vi "hc.vi"(9 "hcUse":string="VARS", 10 "modelName":string="VVV", 11 "Data":dbl[][](array[numeric])) -> ()   [LabVIEW 2014]
uses:
  <vilib>/Analysis/NI_AALBase.lvlib
  <vilib>/Analysis/baseanly.llb/Real A x B.vi
  <vilib>/Analysis/Matrix/NI_Matrix.lvlib
  <vilib>/Analysis/Matrix/Numeric/Conversions/Matrix To Array - RM.vi
  <vilib>/gmath/NI_Gmath.lvlib
panel:
  out "hcPairs":dbl[][](array[numeric])
  in  "Possible Use Names":string[](array[string])=["VARS", "STD", "SPH", "PCS", "PCR", "SVD"]
  in  "Possible Model Names":string[](array[string])=["E", "V", "EII", "VII", "EEE", "VVV"]
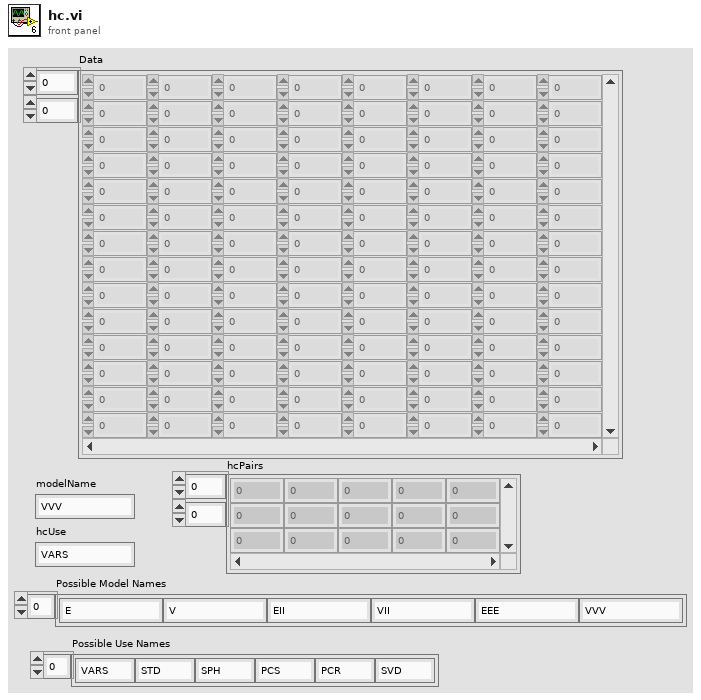
[diagram p1: front panel]
types:
  T1 = typedef "NI_Matrix.lvlib/RealMatrix.ctl" = dbl[][]
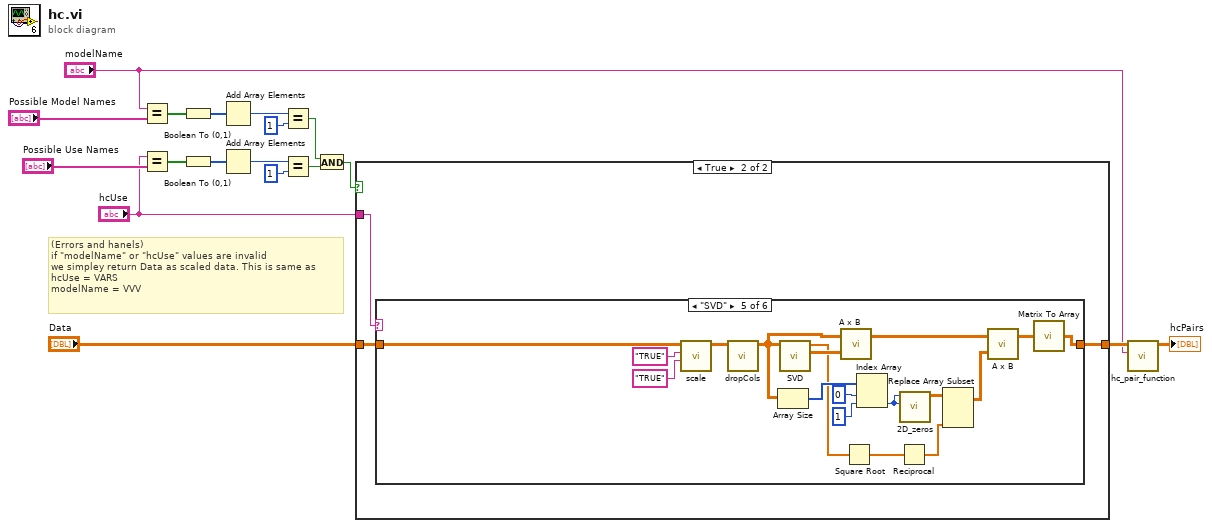
[diagram p0: block diagram]
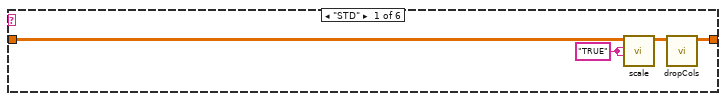
[diagram p3: hidden frame]
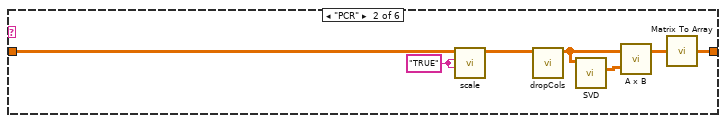
[diagram p4: hidden frame]
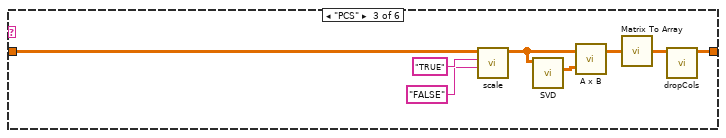
[diagram p5: hidden frame]
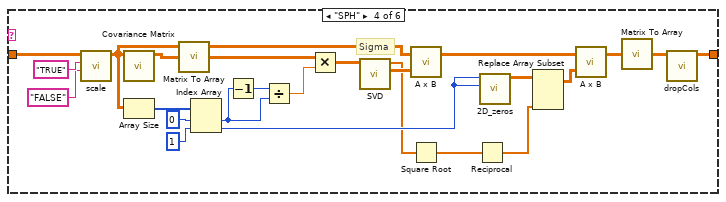
[diagram p6: hidden frame]
diagram:
  # "(Errors and hanels)\nif \"modelName\" or \"hcUse\" values are invalid\nwe simpley return Data as scaled data. This is same as\nhcUse = VARS\nmodelName = VVV"
  n1 = Equal?(x="modelName", y="Possible Model Names") -> (x = y?=w17:bool[])
  n2 = Equal?(x="hcUse", y="Possible Use Names") -> (x = y?=w14:bool[])
  n3 = Boolean To (0,1)(Boolean=w17) -> (0, 1=w16:i16[])
  n4 = Boolean To (0,1)(Boolean=w14) -> (0, 1=w15:i16[])
  n5 = Add Array Elements(numeric array=w16) -> (sum=w12:i16)
  n6 = Add Array Elements(numeric array=w15) -> (sum=w10:i16)
  n7 = Equal?(x=w12, y=i16 1) -> (x = y?=w8:bool)
  n8 = Equal?(x=w10, y=i16 1) -> (x = y?=w7:bool)
  n9 = And(x=w8, y=w7) -> (x .and. y?=w6:bool)
  n10 = case shown="True" w6 {
    tunnel: "Data" -> [w19 w21]
    tunnel: [w19 w20] -> w3
    tunnel: "hcUse" -> [_ w22]
    frame False {
    }
    frame True {
      n11 = case shown="\"SVD\"" w22 {
        tunnel: w21 -> [w26 w33 w38 w65 w68 w84]
        tunnel: [w23 w28 w36 w42 w66 w84] -> w20
        frame "STD" {
          w25 = "TRUE" ("Center")
          n12 = call "scale.vi"("Scale"=w25, "Center"=w25, "data"=w26) -> ("data (scaled)"=w24:dbl[][])  [unwired: 8 in]
          n13 = call "dropCols.vi"("data"=w24) -> ("data (columns dropped)"=w23:dbl[][])  [unwired: 10 in]
        }
        frame "PCR" {
          w32 = "TRUE" ("Center")
          n14 = call "scale.vi"("Scale"=w32, "Center"=w32, "data"=w33) -> ("data (scaled)"=w31:dbl[][])  [unwired: 8 in]
          n15 = call "dropCols.vi"("data"=w31) -> ("data (columns dropped)"=w27:dbl[][])  [unwired: 10 in]
          n16 = call "SVD.vi"("data (scaled)"=w27) -> ("v"=w30:dbl[][])  [unwired: 9 in, 1 out]
          n17 = call-poly <vilib>:"A x B.vi"("B"=w30, "A"=w27) -> ("A x B"=w29:T1)  [unwired: 1 out]
          n18 = call-poly <vilib>:"Matrix To Array.vi"("Real Matrix"=w29) -> ("Real 2D Array"=w28:dbl[][])
        }
        frame "PCS" {
          n19 = call "scale.vi"("Scale"="FALSE" ("Center"), "Center"="TRUE", "data"=w38) -> ("data (scaled)"=w40:dbl[][])  [unwired: 8 in]
          n20 = call "SVD.vi"("data (scaled)"=w40) -> ("v"=w39:dbl[][])  [unwired: 9 in, 1 out]
          n21 = call-poly <vilib>:"A x B.vi"("B"=w39, "A"=w40) -> ("A x B"=w37:T1)  [unwired: 1 out]
          n22 = call-poly <vilib>:"Matrix To Array.vi"("Real Matrix"=w37) -> ("Real 2D Array"=w35:dbl[][])
          n23 = call "dropCols.vi"("data"=w35) -> ("data (columns dropped)"=w36:dbl[][])  [unwired: 10 in]
        }
        frame "SPH" {
          # "Sigma"
          n24 = call "scale.vi"("Scale"="FALSE" ("Center"), "Center"="TRUE", "data"=w65) -> ("data (scaled)"=w54:dbl[][])  [unwired: 8 in]
          n25 = call <vilib>:"Covariance Matrix.vi"("X"=w54) -> ("covariance matrix V"=w56:T1)  [unwired: 9 in, 1 out]
          n26 = Array Size(array=w54) -> (size(s)=w62:i32[])
          n27 = call-poly <vilib>:"Matrix To Array.vi"("Real Matrix"=w56) -> ("Real 2D Array"=w55:dbl[][])
          n28 = Index Array(array=w62, index #1=0 ("index"), index #2=1 ("index")) -> (element #1=w59:i32, element #2=w48:i32)
          n29 = Decrement(x=w59) -> (x-1=w58:i32)
          n30 = Divide(x=w58, y=w59) -> (x/y=w57:dbl)
          n31 = Multiply ("Multiply.vi")(x=w55, y=w57) -> (x*y=w53:dbl[][])
          n32 = call "SVD.vi"("data (scaled)"=w53) -> ("v"=w52:dbl[][], "d"=w46:dbl[])  [unwired: 9 in]
          n33 = call-poly <vilib>:"A x B.vi"("B"=w52, "A"=w54) -> ("A x B"=w51:T1)  [unwired: 1 out]
          n34 = Square Root(x=w46) -> (sqrt(x)=w45:dbl[])
          n35 = Reciprocal(x=w45) -> (1/x=w44:dbl[])
          n36 = call "2D_zeros.vi"("column_number"=w48, "row_number"=w48) -> ("2D_Rand"=w47:dbl[][])  [unwired: 9 in]
          n37 = Replace Array Subset(array=w47, new element=w44) -> (w43:T1)  [unwired: 2 in]
          n38 = call-poly <vilib>:"A x B.vi"("B"=w43, "A"=w51) -> ("A x B"=w50:T1)  [unwired: 1 out]
          n39 = call-poly <vilib>:"Matrix To Array.vi"("Real Matrix"=w50) -> ("Real 2D Array"=w49:dbl[][])
          n40 = call "dropCols.vi"("data"=w49) -> ("data (columns dropped)"=w42:dbl[][])  [unwired: 10 in]
        }
        frame "SVD" {
          n41 = call "scale.vi"("Scale"="TRUE" ("Center"), "Center"="TRUE", "data"=w68) -> ("data (scaled)"=w78:dbl[][])  [unwired: 8 in]
          n42 = call "dropCols.vi"("data"=w78) -> ("data (columns dropped)"=w67:dbl[][])  [unwired: 10 in]
          n43 = Array Size(array=w67) -> (size(s)=w81:i32[])
          n44 = call "SVD.vi"("data (scaled)"=w67) -> ("v"=w77:dbl[][], "d"=w72:dbl[])  [unwired: 9 in]
          n45 = call-poly <vilib>:"A x B.vi"("B"=w77, "A"=w67) -> ("A x B"=w76:T1)  [unwired: 1 out]
          n46 = Square Root(x=w72) -> (sqrt(x)=w71:dbl[])
          n47 = Index Array(array=w81, index #1=0 ("index"), index #2=1 ("index")) -> (element #2=w74:i32)  [unwired: 1 out]
          n48 = Reciprocal(x=w71) -> (1/x=w70:dbl[])
          n49 = call "2D_zeros.vi"("column_number"=w74, "row_number"=w74) -> ("2D_Rand"=w73:dbl[][])  [unwired: 9 in]
          n50 = Replace Array Subset(array=w73, new element=w70) -> (w69:T1)  [unwired: 2 in]
          n51 = call-poly <vilib>:"A x B.vi"("B"=w69, "A"=w76) -> ("A x B"=w75:T1)  [unwired: 1 out]
          n52 = call-poly <vilib>:"Matrix To Array.vi"("Real Matrix"=w75) -> ("Real 2D Array"=w66:dbl[][])
        }
        frame "VARS", Default {
        }
      }
    }
  }
  n53 = call "hc_pair_function.vi"("modelName"="modelName", "data"=w3) -> ("hcPair"=→"hcPairs":dbl[][])  [unwired: 9 in]
